vi "StateMachineExecute.vi"(5 "States finished?":bool=TRUE, 8 "error in (no error)":errorcluster, 11 "StateMachine in":refnum<class "StateMachine.lvclass">) -> (0 "error out":errorcluster, 2 "output cluster":T1, 3 "StateMachine out":refnum<class "StateMachine.lvclass">)   [LabVIEW 2018, in "StateMachine.lvclass"]
uses:
  StateMachine.lvclass
  StateMachine.lvclass/StateMachine.ctl
  <vilib>/Rock Robotics/WPI/ThirdParty/Phoenix-LabVIEW/Motor Controller/Controls/CTRE_Phoenix_MotorControl_ControlMode.ctl
  <vilib>/Rock Robotics/WPI/Solenoid/WPI_SolenoidSetEnum.vi
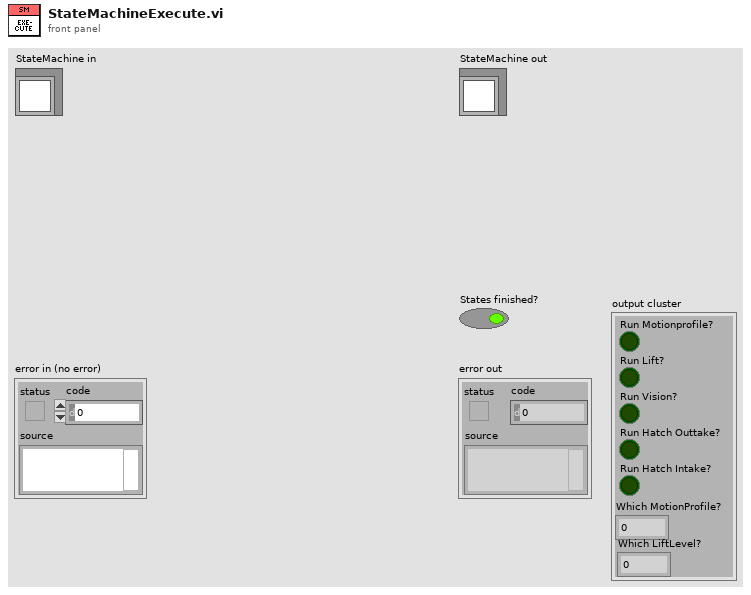
[diagram p1: front panel]
types:
  T1 = cluster{"Run Motionprofile?":bool, "Run Lift?":bool, "Run Vision?":bool, "Run Hatch Outtake?":bool, "Run Hatch Intake?":bool, "Which MotionProfile?":dbl, "Which LiftLevel?":dbl}
  T2 = cluster{"Run Motionprofile?":bool, "Run Lift?":bool, "Run Vision?":bool, "Run Hatch Outtake?":bool, "Run Hatch Intake?":bool, "Which MotionProfile?":i32, "Which LiftLevel?":i32}
  T3 = typedef "CTRE_Phoenix_MotorControl_ControlMode.ctl" = u16
  T4 = typedef "WPI_MotorControlDeviceRef.ctl" = cluster{"DeviceStatus":errorcluster, "Type":T5, "PWM":cluster{"PWM Channel":T6, "DeadBand":T7}, "CAN":cluster{"Device Number":u8, "SetOutput VI Ref":variant, "GetOutput VI Ref":variant, "Enable VI Ref":variant, "Disable VI Ref":variant, "Data":variant}, "Invert":bool, "DIO PWM":cluster{"PWM \"Enable\" Channel":T6, "DIOChannel":T8, "PWM Rate":dbl}}
  T5 = typedef "WPI_MotorControlType.ctl" = enum16{"PWM", "CAN", "DIO PWM"}
  T6 = typedef "FPGA_DIOPWMChannel.ctl" = enum8{"PWM 0", "PWM 1", "PWM 2", "PWM 3", "PWM 4", "PWM 5", "PWM 6", "PWM 7", "PWM 8", "PWM 9", "PWM MXP 0", "PWM MXP 1", "PWM MXP 2", "PWM MXP 3", "PWM MXP 4", "PWM MXP 5", "PWM MXP 6", "PWM MXP 7", "PWM MXP 8", "PWM MXP 9", "Invalid"}
  T7 = typedef "WPI_PWMDeadband.ctl" = cluster{"Name":string, "maxPositivePwm":i32, "minPositivePwm":i32, "centerPwm":i32, "maxNegativePwm":i32, "minNegativePwm":i32, "angularRange":u16}
  T8 = typedef "FPGA_DIOChannel.ctl" = enum8{"DIO 0", "DIO 1", "DIO 2", "DIO 3", "DIO 4", "DIO 5", "DIO 6", "DIO 7", "DIO 8", "DIO 9", "DIO MXP 0", "DIO MXP 1", "DIO MXP 2", "DIO MXP 3", "DIO MXP 4", "DIO MXP 5", "DIO MXP 6", "DIO MXP 7", "DIO MXP 8", "DIO MXP 9", "DIO MXP 10", "DIO MXP 11", "DIO MXP 12", "DIO MXP 13", "DIO MXP 14", "DIO MXP 15", "SPI Port CS1", "SPI Port CS2", "SPI Port CS3", "SPI Port MISO", "SPI Port MOSI", "Invalid"}
  T9 = typedef "WPI_SolenoidDevRef.ctl" = cluster{"DevStatus":errorcluster, "Pneumatics Control Module":u8, "Forward Solenoid Channel":T10, "Reverse Solenoid Channel":T10}
  T10 = typedef "WPI_SolenoidChannel.ctl" = enum8{"Solenoid 0", "Solenoid 1", "Solenoid 2", "Solenoid 3", "Solenoid 4", "Solenoid 5", "Solenoid 6", "Solenoid 7", "Invalid"}
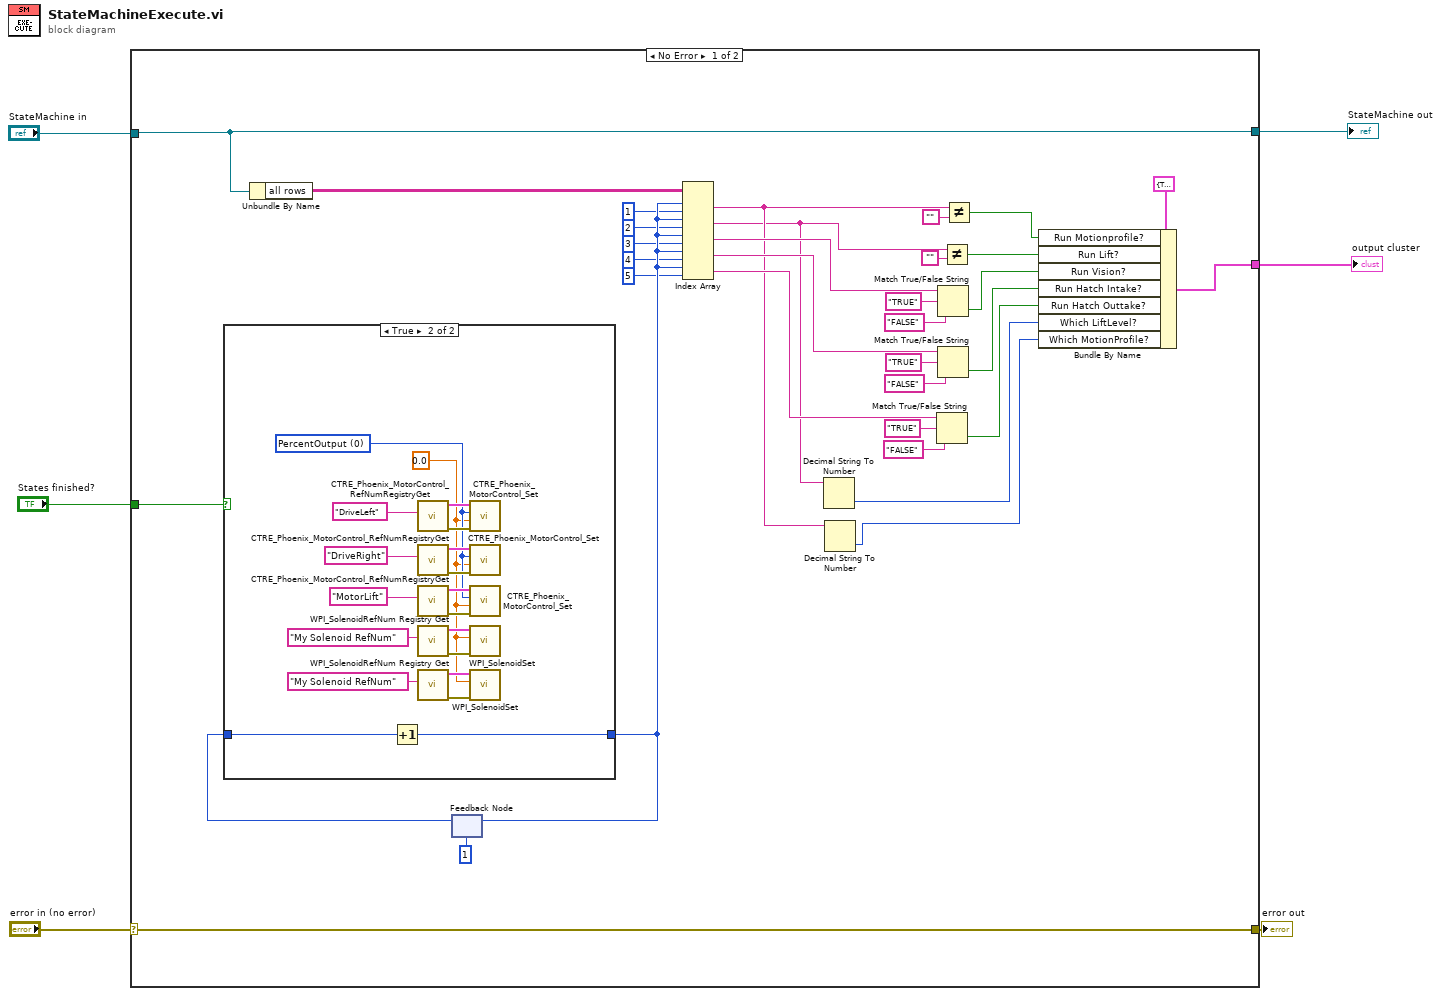
[diagram p0: block diagram]
diagram:
  n1 = case shown="No Error" "error in (no error)" {
    selector: "error in (no error)" -> [w40 w62]
    tunnel: [w40 w62] -> w5
    tunnel: [w12 w61] -> w3
    tunnel: "StateMachine in" -> [w12 w61]
    tunnel: [w13 _] -> w2
    tunnel: "States finished?" -> [w9 _]
    frame No Error {
      n2 = Unbundle By Name(w12) -> ("all rows"=w39:string[][])
      n3 = feedback #1(1) -> (w38:i32)
      n4 = case shown="True" w9 {
        tunnel: w38 -> [w41 w43]
        tunnel: [w41 w42] -> w36
        frame False {
        }
        frame True {
          w44 = 0.0 ("Output")
          w45 = T3 0 items=["PercentOutput"=0, "Position"=1, "Velocity"=2, "Current"=3, "Follower"=5, "MotionProfile"=6, "MotionMagic"=7, "MotionProfileArc"=10, "Disabled"=15] ("Control Mode")
          n5 = Increment(x=w43) -> (x+1=w42:i32)
          n6 = call <vilib>:"CTRE_Phoenix_MotorControl_RefNumRegistryGet.vi"("refnum name"="DriveLeft") -> ("error out"=w60:errorcluster, "PhoenixMotorControlDevRef"=w59:T4)  [unwired: 9 in]
          n7 = call <vilib>:"CTRE_Phoenix_MotorControl_RefNumRegistryGet.vi"("refnum name"="DriveRight") -> ("error out"=w57:errorcluster, "PhoenixMotorControlDevRef"=w56:T4)  [unwired: 9 in]
          n8 = call <vilib>:"CTRE_Phoenix_MotorControl_RefNumRegistryGet.vi"("refnum name"="MotorLift") -> ("error out"=w54:errorcluster, "PhoenixMotorControlDevRef"=w53:T4)  [unwired: 9 in]
          n9 = call <vilib>:"WPI_SolenoidRefNum Registry Get.vi"("refnum name"="My Solenoid RefNum") -> ("error out"=w51:errorcluster, "SolenoidDevRef"=w50:T9)  [unwired: 9 in]
          n10 = call <vilib>:"WPI_SolenoidRefNum Registry Get.vi"("refnum name"="My Solenoid RefNum") -> ("error out"=w48:errorcluster, "SolenoidDevRef"=w47:T9)  [unwired: 9 in]
          n11 = call <vilib>:"CTRE_Phoenix_MotorControl_Set.vi"("error in (no error)"=w60, "Output"=w44, "Control Mode"=w45, "PhoenixMotorControlDevRef"=w59) -> ()  [unwired: 6 in, 2 out]
          n12 = call <vilib>:"CTRE_Phoenix_MotorControl_Set.vi"("error in (no error)"=w57, "Output"=w44, "Control Mode"=w45, "PhoenixMotorControlDevRef"=w56) -> ()  [unwired: 6 in, 2 out]
          n13 = call <vilib>:"CTRE_Phoenix_MotorControl_Set.vi"("error in (no error)"=w54, "Output"=w44, "Control Mode"=w45, "PhoenixMotorControlDevRef"=w53) -> ()  [unwired: 6 in, 2 out]
          n14 = call-poly <vilib>:"WPI_SolenoidSet.vi"("error in (no error)"=w51, "Value"=w44, "SolenoidDevRef"=w50) -> ()  [unwired: 7 in, 2 out]
          n15 = call-poly <vilib>:"WPI_SolenoidSet.vi"("error in (no error)"=w48, "Value"=w44, "SolenoidDevRef"=w47) -> ()  [unwired: 7 in, 2 out]
        }
      }
      n16 = feedback-in #1(w36) -> ()
      n17 = Index Array(array=w39, index (row) #1=w36, index (col) #1=1 ("disabled index (col)"), index (row) #2=w36, index (col) #2=2 ("disabled index (col)"), index (row) #3=w36, index (col) #3=3 ("disabled index (col)"), index (row) #4=w36, index (col) #4=4 ("disabled index (col)"), index (row) #5=w36, index (col) #5=5 ("disabled index (col)")) -> (element #1=w11:string, element #2=w8:string, element #3=w30:string, element #4=w23:string, element #5=w22:string)
      n18 = Decimal String To Number(string=w8) -> (number=w7:i32)  [unwired: 2 in, 1 out]
      n19 = Decimal String To Number(string=w11) -> (number=w10:i32)  [unwired: 2 in, 1 out]
      n20 = Match True/False String(2:"FALSE" ("false string"), 3:"TRUE" ("true string"), 4:w22) -> (0:w14:bool)  [unwired: 1 out]
      n21 = Match True/False String(2:"FALSE" ("false string"), 3:"TRUE" ("true string"), 4:w30) -> (0:w16:bool)  [unwired: 1 out]
      n22 = Match True/False String(2:"FALSE" ("false string"), 3:"TRUE" ("true string"), 4:w23) -> (0:w15:bool)  [unwired: 1 out]
      n23 = Not Equal?(x=w8, y="") -> (x != y?=w17:bool)
      n24 = Not Equal?(x=w11, y="") -> (x != y?=w18:bool)
      n25 = Bundle By Name(cluster=T2 {"Run Motionprofile?"=TRUE, "Run Lift?"=TRUE, "Run Vision?"=TRUE, "Run Hatch Outtake?"=TRUE, "Run Hatch Intake?"=TRUE, "Which MotionProfile?"=0, "Which LiftLevel?"=0}, "Run Motionprofile?"=w18, "Run Lift?"=w17, "Run Vision?"=w16, "Run Hatch Intake?"=w15, "Run Hatch Outtake?"=w14, "Which LiftLevel?"=w7, "Which MotionProfile?"=w10) -> (w13:T2)
    }
    frame Error {
    }
  }
  "error out" <- w5
  "StateMachine out" <- w3
  "output cluster" <- w2
